vi "gate percent to width.vi"(2 "Trigger Freq":dbl[unit], 3 "Gate %":dbl) -> (1 "Gate width":dbl[unit])   [LabVIEW 2011]
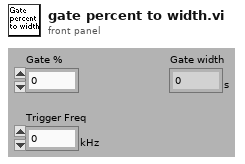
[diagram p1: front panel]
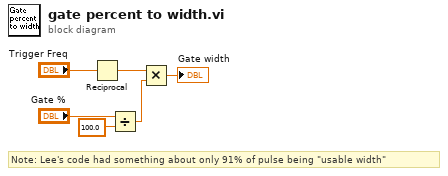
[diagram p0: block diagram]
diagram:
  # "Note: Lee's code had something about only 91% of pulse being \"usable width\""
  n1 = Reciprocal(x="Trigger Freq") -> (1/x=w1:dbl[unit])
  n2 = Divide(x="Gate %", y=100.0) -> (x/y=w5:dbl)
  n3 = Multiply(x=w1, y=w5) -> (x*y=→"Gate width":dbl[unit])
